vi "DisplayArrayCreator.vi"(9 "Number of Points":i32, 10 "Location of the Trigger":i32, 11 "Input Y Values":dbl[](array[numeric])) -> (1 "Valid?":bool, 3 "Output Y Values":dbl[](array[numeric]))   [LabVIEW 2014]
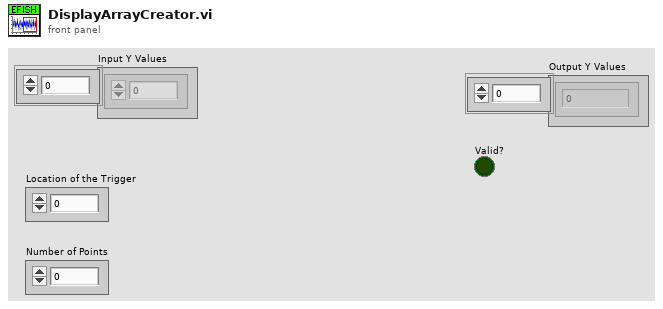
[diagram p1: front panel]
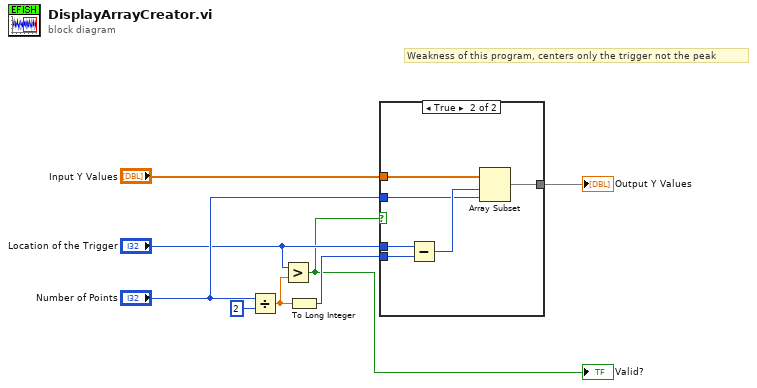
[diagram p0: block diagram]
diagram:
  # "Weakness of this program, centers only the trigger not the peak"
  n1 = Divide(x="Number of Points", y=2) -> (x/y=w2:dbl)
  n2 = Greater?(x="Location of the Trigger", y=w2) -> (0:w1:bool)
  "Valid?" <- w1
  n3 = To Long Integer(number=w2) -> (32bit integer=w6:i32)
  n4 = case shown="True" w1 {
    tunnel: "Input Y Values" -> [w9 w15]
    tunnel: w6 -> [_ w14]
    tunnel: "Number of Points" -> [_ w12]
    tunnel: [w9 w11] -> w4
    tunnel: "Location of the Trigger" -> [_ w10]
    frame False {
    }
    frame True {
      n5 = Subtract(x=w10, y=w14) -> (x-y=w13:i32)
      n6 = Array Subset(array=w15, index=w13, length=w12) -> (w11:dbl[])
    }
  }
  "Output Y Values" <- w4
